vi "Write TimeoutTactic.vi"(8 "error in (no error)":errorcluster, 10 "TimeoutTactic":refnum<class "TimeoutTactic.lvclass">, 11 "Tacticbook in":refnum<class "Tacticbook.lvclass">) -> (0 "error out":errorcluster, 3 "Tacticbook out":refnum<class "Tacticbook.lvclass">)   [LabVIEW 2023, in "Tacticbook.lvclass"]
uses:
  Tacticbook.lvclass
  TimeoutTactic_class/TimeoutTactic.lvclass
  Tacticbook.lvclass/Tacticbook.ctl
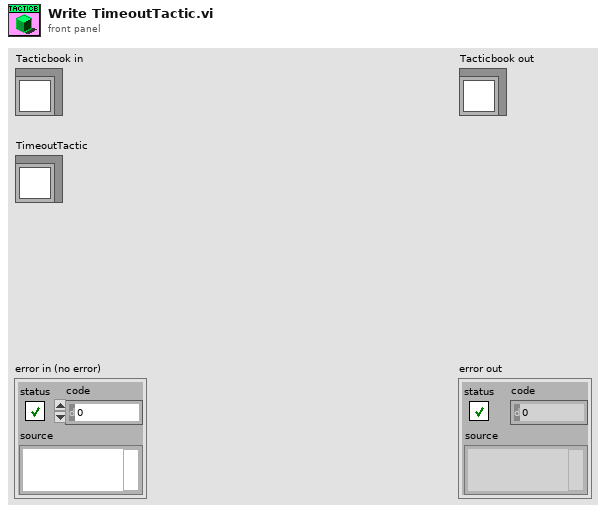
[diagram p1: front panel]
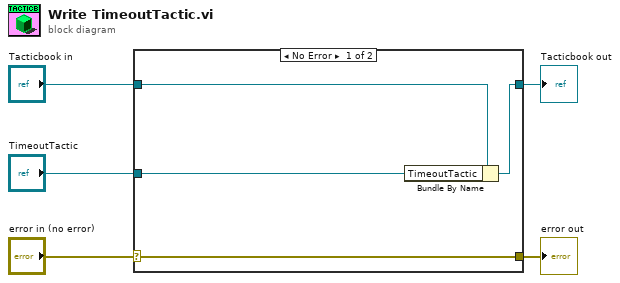
[diagram p0: block diagram]
diagram:
  n1 = case shown="No Error" "error in (no error)" {
    selector: "error in (no error)" -> [w9 w10]
    tunnel: [w9 w10] -> w4
    tunnel: [w7 w11] -> w2
    tunnel: "Tacticbook in" -> [w8 w11]
    tunnel: "TimeoutTactic" -> [w6 _]
    frame No Error {
      n2 = Bundle By Name(cluster=w8, "TimeoutTactic"=w6) -> (w7:refnum<class "Tacticbook.lvclass">)
    }
    frame Error {
    }
  }
  "error out" <- w4
  "Tacticbook out" <- w2
